vi "Acquire Data from 1 BPM.vi"(4 "error in (no error)":errorcluster, 7 "VISA resource in":refnum<visa-resource-name>) -> (0 "error out":errorcluster, 3 "VISA resource out":refnum<visa-resource-name>)   [LabVIEW 2015]
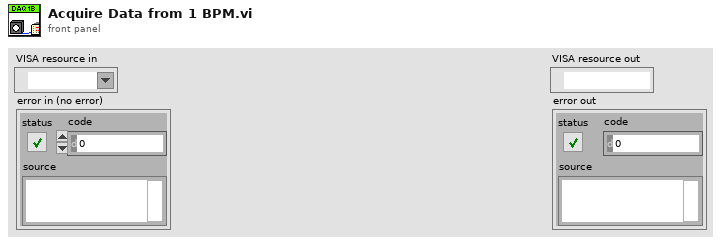
[diagram p1: front panel]
types:
  T1 = enum16{"Channel 1", "Channel 2", "Channel 3", "Channel 4"}[]
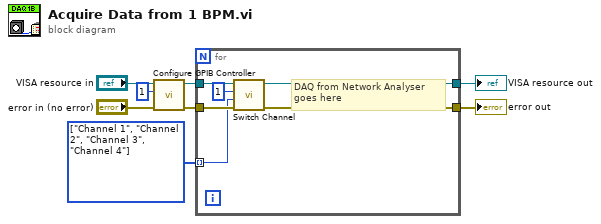
[diagram p0: block diagram]
diagram:
  w8 = T1 [enum."Channel 1", enum."Channel 2", enum."Channel 3", enum."Channel 4"] items=["Channel 1", "Channel 2", "Channel 3", "Channel 4"] ("Channel to Select")
  n1 = call "Configure GPIB Controller.vi"("error in (no error)"="error in (no error)", "Address"=u32 1, "VISA Refnum in"="VISA resource in") -> ("error out"=w4:errorcluster, "VISA Refnum out"=w5:refnum<visa-resource-name>)  [unwired: 7 in]
  n2 = for {
    tunnel: w5 -> [w14]
    tunnel: w4 -> [w12]
    tunnel: w8 -> [w11] mode=indexing
    tunnel: [w10] -> w7
    tunnel: [w9] -> w6
    # "DAQ from Network Analyser\ngoes here"
    n3 = call "Switch Channel.vi"("error in (no error)"=w12, "Channel to select"=w11, "Card Number"=u8 1, "VISA resource in"=w14) -> ("error out"=w9:errorcluster, "VISA resource out"=w10:refnum<visa-resource-name>)  [unwired: 2 in]
  }
  "VISA resource out" <- w7
  "error out" <- w6
